vi "CTRE_CANTalonSRX_ConfigEnabledLimits.vi"(0 "CAN Talon SRX Ref":T1={"DeviceStatus"={"status"=FALSE, "code"=0, "source"=""}, "Type"=enum."PWM", "PWM"={"PWM Channel"=enum."PWM 1", "DeadBand"={"Name"="", "maxPositivePwm"=0, "minPositivePwm"=0, "centerPwm"=0, "maxNegativePwm"=0, "minNegativePwm"=0, "angularRange"=0}}, "CAN"={"Device Number"=0, "SetOutput VI Ref"=variant(enum8{"Percent VBus", "Current", "Speed", "Position", "Voltage"} enum."Percent VBus"), "GetOutput VI Ref"=variant(refnum<k1> refnum), "Enable VI Ref"=variant(dbl 12.0), "Disable VI Ref"=variant(enum8{"Percent VBus", "Speed", "Position", "Slave", "Unchanged / Invalid", "Voltage Compensation", "Current", "Motion Profile"} enum."Percent VBus"), "Data"=variant}, "Invert"=FALSE}, 5 "Override Limit Switches":bool, 7 "Forward Limit Switch Enable":bool=TRUE, 9 "Reverse Limit Switch Enable":bool=TRUE, 11 "error in (no error)":errorcluster, 12 "Forward Soft Limit Enable":bool, 13 "Reverse Soft Limit Enable":bool) -> (4 "CAN Talon SRX Ref":T1={"DeviceStatus"={"status"=FALSE, "code"=0, "source"=""}, "Type"=enum."PWM", "PWM"={"PWM Channel"=enum."PWM 1", "DeadBand"={"Name"="", "maxPositivePwm"=0, "minPositivePwm"=0, "centerPwm"=0, "maxNegativePwm"=0, "minNegativePwm"=0, "angularRange"=0}}, "CAN"={"Device Number"=0, "SetOutput VI Ref"=variant(enum8{"Percent VBus", "Current", "Speed", "Position", "Voltage"} enum."Percent VBus"), "GetOutput VI Ref"=variant(refnum<k1> refnum), "Enable VI Ref"=variant(dbl 12.0), "Disable VI Ref"=variant(enum8{"Percent VBus", "Speed", "Position", "Slave", "Unchanged / Invalid", "Voltage Compensation", "Current", "Motion Profile"} enum."Percent VBus"), "Data"=variant}, "Invert"=FALSE}, 15 "error out":errorcluster)   [LabVIEW 2016]
doc: "Configure the enable state of the hardware limit switches and the soft limits."
uses:
  <vilib>/Rock Robotics/WPI/MotorControl/WPI_MotorControlDeviceRef.ctl
  <vilib>/Rock Robotics/WPI/MotorControl/WPI_MotorControlType.ctl
  <vilib>/Rock Robotics/SystemInterfaces/DIO/FPGA_DIOPWMChannel.ctl
  <vilib>/Rock Robotics/WPI/PWM/WPI_PWMDeadband.ctl
  <vilib>/Rock Robotics/WPI/ThirdParty/CanMotor/CTRLib-LV-TalonSRX/CTRE_CANTalonSRX_Params.ctl
  <vilib>/Rock Robotics/WPI/ThirdParty/CanMotor/CTRLib-LV-TalonSRX/CTRE_CANTalonSRX_UsageTypes.ctl
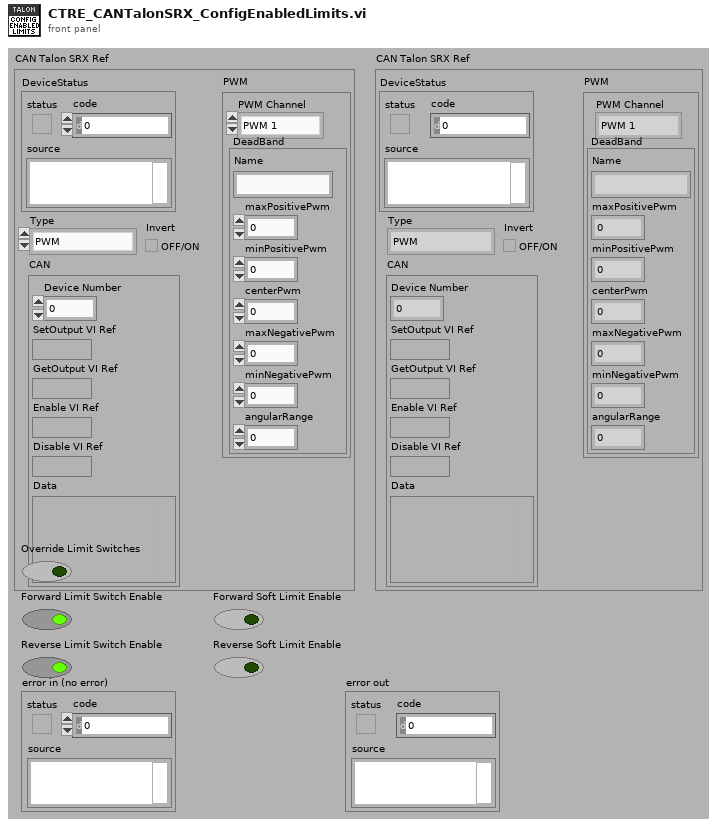
[diagram p1: front panel]
types:
  T1 = typedef "WPI_MotorControlDeviceRef.ctl" = cluster{"DeviceStatus":errorcluster, "Type":T2, "PWM":cluster{"PWM Channel":T3, "DeadBand":T4}, "CAN":cluster{"Device Number":u8, "SetOutput VI Ref":variant, "GetOutput VI Ref":variant, "Enable VI Ref":variant, "Disable VI Ref":variant, "Data":variant}, "Invert":bool}
  T2 = typedef "WPI_MotorControlType.ctl" = enum16{"PWM", "CAN"}
  T3 = typedef "FPGA_DIOPWMChannel.ctl" = enum8{"PWM 0", "PWM 1", "PWM 2", "PWM 3", "PWM 4", "PWM 5", "PWM 6", "PWM 7", "PWM 8", "PWM 9", "PWM MXP 0", "PWM MXP 1", "PWM MXP 2", "PWM MXP 3", "PWM MXP 4", "PWM MXP 5", "PWM MXP 6", "PWM MXP 7", "PWM MXP 8", "PWM MXP 9", "Invalid"}
  T4 = typedef "WPI_PWMDeadband.ctl" = cluster{"Name":string, "maxPositivePwm":i32, "minPositivePwm":i32, "centerPwm":i32, "maxNegativePwm":i32, "minNegativePwm":i32, "angularRange":u16}
  T5 = typedef "CTRE_CANTalonSRX_Params.ctl" = u8
  T6 = typedef "CTRE_CANTalonSRX_UsageTypes.ctl" = u32
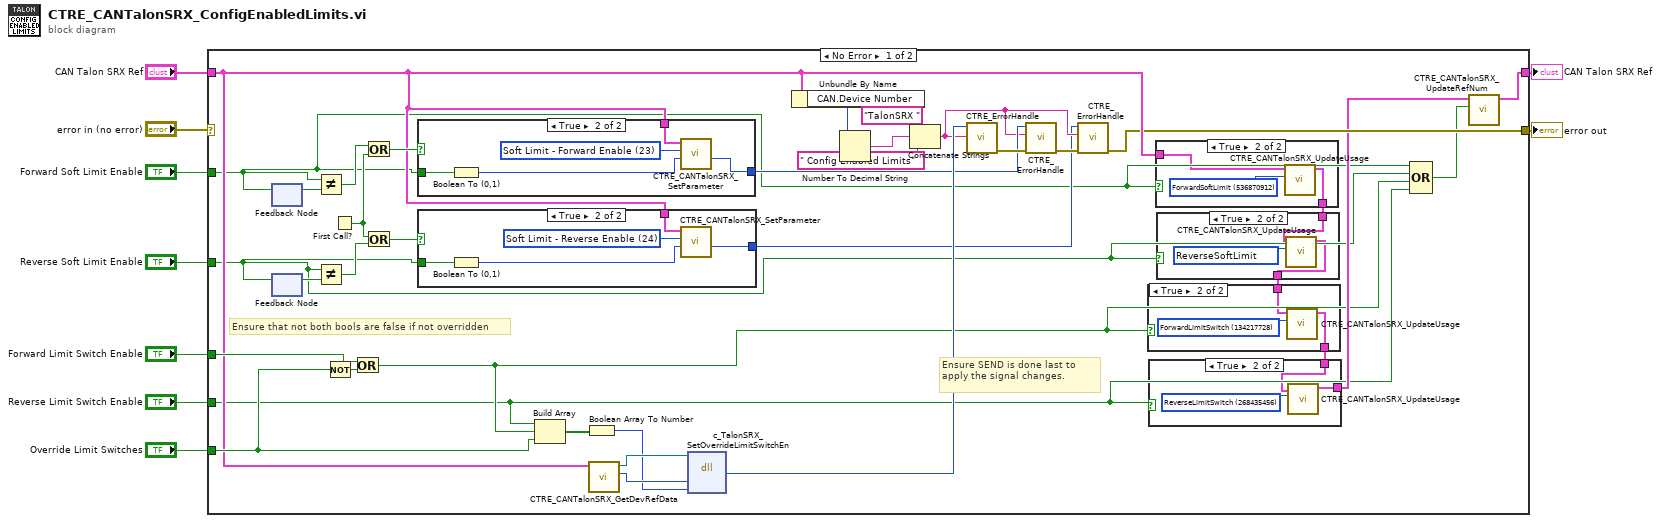
[diagram p0: block diagram]
diagram:
  n1 = case shown="No Error" "error in (no error)" {
    selector: "error in (no error)" -> [_ w73]
    tunnel: [w20 w73] -> w9
    tunnel: [w19 w72] -> w7
    tunnel: "CAN Talon SRX Ref" -> [w27 w72]
    tunnel: "Reverse Soft Limit Enable" -> [w13 _]
    tunnel: "Forward Soft Limit Enable" -> [w14 _]
    tunnel: "Reverse Limit Switch Enable" -> [w11 _]
    tunnel: "Forward Limit Switch Enable" -> [w37 _]
    tunnel: "Override Limit Switches" -> [w36 _]
    frame No Error {
      # "Ensure that not both bools are false if not overridden"
      # "Ensure SEND is done last to apply the signal changes."
      n2 = feedback #1() -> (w41:bool)  [unwired: 1 in]
      n3 = feedback-in #1(w14) -> ()
      n4 = feedback-in #2(w13) -> ()
      n5 = feedback #2() -> (w45:bool)  [unwired: 1 in]
      n6 = Not Equal?(x=w14, y=w41) -> (x != y?=w42:bool)
      n7 = Not Equal?(x=w13, y=w45) -> (x != y?=w43:bool)
      n8 = Not(x=w36) -> (.not. x?=w38:bool)
      n9 = First Call?() -> (First Call?: T/F=w40:bool)
      n10 = Or(x=w37, y=w38) -> (x .or. y?=w12:bool)
      n11 = Or(x=w42, y=w40) -> (x .or. y?=w39:bool)
      n12 = Or(x=w40, y=w43) -> (x .or. y?=w44:bool)
      n13 = case shown="True" w39 {
        tunnel: w14 -> [_ w65]
        tunnel: w27 -> [_ w63]
        tunnel: [_ w62] -> w24
        frame False {
        }
        frame True {
          w66 = T5 23 items=["Slot 0 - P"=1, "Slot 0 - I"=2, "Slot 0 - D"=3, "Slot 0 - F"=4, "Slot 0 - I Zone"=5, "Slot 0 - Ramp Rate"=6, "Slot 1 - P"=11, "Slot 1 - I"=12, "Slot 1 - D"=13, "Slot 1 - F"=14, "Slot 1 - I Zone"=15, "Slot 1 - Ramp Rate"=16, "Soft Limit - Forward"=21, "Soft Limit - Reverse"=22, "Soft Limit - Forward Enable"=23, "Soft Limit - Reverse Enable"=24, "On Boot - Brake Mode"=31, "On Boot - Limit Normally Closed - Forward"=32, "On Boot - Limit Normally Closed - Reverse"=33, "On Boot - Limit Disabled - Forward"=34, "On Boot - Limit Disabled - Reverse"=35, "Fault - Over Temp"=41, "Fault - Under Voltage"=42, "Fault - Forward Limit"=43, "Fault - Reverse Limit"=44, "Fault - Hardware Failure"=45, "Fault - Forward Soft Limit"=46, "Fault - Reverse Soft Limit"=47, "Sticky Fault - Over Temp"=48, "Sticky Fault - Under Voltage"=49, "Sticky Fault - Forward Limit"=50, "Sticky Fault - Reverse Limit"=51, "Sticky Fault - Forward Soft Limit"=52, "Sticky Fault - Reverse Soft Limit"=53, "Applied Throttle"=61, "Closed-Loop Error"=62, "Select Feedback Device"=63, "Reverse Closed-Loop Output"=64, "Mode Select"=65, "Profile Slot Select"=66, "Ramp Throttle"=67, "Reverse Feedback Sensor"=68, "Limit Switch Enabled"=69, "Limit Switch Closed - Forward"=70, "Limit Switch Closed - Reverse"=71, "Sensor Position"=73, "Sensor Velocity"=74, "Current"=75, "Brake is Enabled"=76, "Encoder Position"=77, "Encoder Velocity"=78, "Encoder Index Rise Events"=79, "Encoder A Pin State"=80, "Encoder B Pin State"=81, "Encoder Index Pin State"=82, "Analog In with Overflow"=83, "Analog In Velocity"=84, "Temperature"=85, "Battery Voltage"=86, "Reset Count"=87, "Reset Flags"=88, "Firmware Version"=89, "Settings Changed"=90] ("Parameter")
          n14 = Boolean To (0,1)(Boolean=w65) -> (0, 1=w64:i16)
          n15 = call <vilib>:"CTRE_CANTalonSRX_SetParameter.vi"("Value"=w64, "Parameter"=w66, "CAN Talon SRX Ref"=w63) -> ("Error Code"=w62:i32)  [unwired: 6 in, 2 out]
        }
      }
      n16 = case shown="True" w44 {
        tunnel: w13 -> [_ w70]
        tunnel: w27 -> [_ w68]
        tunnel: [_ w67] -> w21
        frame False {
        }
        frame True {
          w71 = T5 24 items=["Slot 0 - P"=1, "Slot 0 - I"=2, "Slot 0 - D"=3, "Slot 0 - F"=4, "Slot 0 - I Zone"=5, "Slot 0 - Ramp Rate"=6, "Slot 1 - P"=11, "Slot 1 - I"=12, "Slot 1 - D"=13, "Slot 1 - F"=14, "Slot 1 - I Zone"=15, "Slot 1 - Ramp Rate"=16, "Soft Limit - Forward"=21, "Soft Limit - Reverse"=22, "Soft Limit - Forward Enable"=23, "Soft Limit - Reverse Enable"=24, "On Boot - Brake Mode"=31, "On Boot - Limit Normally Closed - Forward"=32, "On Boot - Limit Normally Closed - Reverse"=33, "On Boot - Limit Disabled - Forward"=34, "On Boot - Limit Disabled - Reverse"=35, "Fault - Over Temp"=41, "Fault - Under Voltage"=42, "Fault - Forward Limit"=43, "Fault - Reverse Limit"=44, "Fault - Hardware Failure"=45, "Fault - Forward Soft Limit"=46, "Fault - Reverse Soft Limit"=47, "Sticky Fault - Over Temp"=48, "Sticky Fault - Under Voltage"=49, "Sticky Fault - Forward Limit"=50, "Sticky Fault - Reverse Limit"=51, "Sticky Fault - Forward Soft Limit"=52, "Sticky Fault - Reverse Soft Limit"=53, "Applied Throttle"=61, "Closed-Loop Error"=62, "Select Feedback Device"=63, "Reverse Closed-Loop Output"=64, "Mode Select"=65, "Profile Slot Select"=66, "Ramp Throttle"=67, "Reverse Feedback Sensor"=68, "Limit Switch Enabled"=69, "Limit Switch Closed - Forward"=70, "Limit Switch Closed - Reverse"=71, "Sensor Position"=73, "Sensor Velocity"=74, "Current"=75, "Brake is Enabled"=76, "Encoder Position"=77, "Encoder Velocity"=78, "Encoder Index Rise Events"=79, "Encoder A Pin State"=80, "Encoder B Pin State"=81, "Encoder Index Pin State"=82, "Analog In with Overflow"=83, "Analog In Velocity"=84, "Temperature"=85, "Battery Voltage"=86, "Reset Count"=87, "Reset Flags"=88, "Firmware Version"=89, "Settings Changed"=90] ("Parameter")
          n17 = Boolean To (0,1)(Boolean=w70) -> (0, 1=w69:i16)
          n18 = call <vilib>:"CTRE_CANTalonSRX_SetParameter.vi"("Value"=w69, "Parameter"=w71, "CAN Talon SRX Ref"=w68) -> ("Error Code"=w67:i32)  [unwired: 6 in, 2 out]
        }
      }
      n19 = Build Array(w11, w12, w36) -> (w33:bool[])
      n20 = Boolean Array To Number(Boolean array=w33) -> (number=w32:u8)
      n21 = call <vilib>:"CTRE_CANTalonSRX_GetDevRefData.vi"("MotorControlDevRef"=w27) -> ("handle"=w34:u64, "Library"=w35:path)  [unwired: 6 in, 3 out]
      n22 = dll-call lib="?" fn="c_TalonSRX_SetOverrideLimitSwitchEn"(path in=w35, "handle"=w34, "param"=w32) -> ("return type"=w26:i32)  [unwired: 4 in, 2 out]
      n23 = Unbundle By Name(w27) -> ("CAN.Device Number"=w28:u8)
      n24 = Number To Decimal String(number=w28) -> (decimal integer string=w30:string)  [unwired: 1 in]
      n25 = Concatenate Strings("TalonSRX " ("string"), w30, " Config Enabled Limits" ("string")) -> (w22:string)
      n26 = call <vilib>:"CTRE_ErrorHandle.vi"("origin"=w22, "code"=w26) -> ("error out"=w25:errorcluster)  [unwired: 9 in]
      n27 = call <vilib>:"CTRE_ErrorHandle.vi"("error in"=w25, "origin"=w22, "code"=w24) -> ("error out"=w23:errorcluster)  [unwired: 8 in]
      n28 = call <vilib>:"CTRE_ErrorHandle.vi"("error in"=w23, "origin"=w22, "code"=w21) -> ("error out"=w20:errorcluster)  [unwired: 8 in]
      n29 = case shown="True" w14 {
        tunnel: w27 -> [w58 w61]
        tunnel: [w58 w59] -> w18
        frame False {
        }
        frame True {
          w60 = T6 536870912 items=["Default"=0, "PercentVbus"=1, "Position"=2, "Speed"=4, "Current"=8, "Voltage"=16, "Follower"=32, "MotionProfile"=64, "MotionMagic"=128, "VRampRate"=4194304, "CurrentLimit"=8388608, "ZeroSensorI"=16777216, "ZeroSensorF"=33554432, "ZeroSensorR"=67108864, "ForwardLimitSwitch"=134217728, "ReverseLimitSwitch"=268435456, "ForwardSoftLimit"=536870912, "ReverseSoftLimit"=1073741824, "MultiProfile"=2147483648] ("Usage")
          n30 = call <vilib>:"CTRE_CANTalonSRX_UpdateUsage.vi"("Usage"=w60, "CAN Talon SRX Ref"=w61) -> ("CAN Talon SRX"=w59:T1)  [unwired: 8 in, 1 out]
        }
      }
      n31 = case shown="True" w13 {
        tunnel: w18 -> [w54 w56]
        tunnel: [w54 w55] -> w17
        frame False {
        }
        frame True {
          w57 = T6 1073741824 items=["Default"=0, "PercentVbus"=1, "Position"=2, "Speed"=4, "Current"=8, "Voltage"=16, "Follower"=32, "MotionProfile"=64, "MotionMagic"=128, "VRampRate"=4194304, "CurrentLimit"=8388608, "ZeroSensorI"=16777216, "ZeroSensorF"=33554432, "ZeroSensorR"=67108864, "ForwardLimitSwitch"=134217728, "ReverseLimitSwitch"=268435456, "ForwardSoftLimit"=536870912, "ReverseSoftLimit"=1073741824, "MultiProfile"=2147483648] ("Usage")
          n32 = call <vilib>:"CTRE_CANTalonSRX_UpdateUsage.vi"("Usage"=w57, "CAN Talon SRX Ref"=w56) -> ("CAN Talon SRX"=w55:T1)  [unwired: 8 in, 1 out]
        }
      }
      n33 = case shown="True" w12 {
        tunnel: w17 -> [w50 w52]
        tunnel: [w50 w51] -> w16
        frame False {
        }
        frame True {
          w53 = T6 134217728 items=["Default"=0, "PercentVbus"=1, "Position"=2, "Speed"=4, "Current"=8, "Voltage"=16, "Follower"=32, "MotionProfile"=64, "MotionMagic"=128, "VRampRate"=4194304, "CurrentLimit"=8388608, "ZeroSensorI"=16777216, "ZeroSensorF"=33554432, "ZeroSensorR"=67108864, "ForwardLimitSwitch"=134217728, "ReverseLimitSwitch"=268435456, "ForwardSoftLimit"=536870912, "ReverseSoftLimit"=1073741824, "MultiProfile"=2147483648] ("Usage")
          n34 = call <vilib>:"CTRE_CANTalonSRX_UpdateUsage.vi"("Usage"=w53, "CAN Talon SRX Ref"=w52) -> ("CAN Talon SRX"=w51:T1)  [unwired: 8 in, 1 out]
        }
      }
      n35 = case shown="True" w11 {
        tunnel: w16 -> [w46 w48]
        tunnel: [w46 w47] -> w15
        frame False {
        }
        frame True {
          w49 = T6 268435456 items=["Default"=0, "PercentVbus"=1, "Position"=2, "Speed"=4, "Current"=8, "Voltage"=16, "Follower"=32, "MotionProfile"=64, "MotionMagic"=128, "VRampRate"=4194304, "CurrentLimit"=8388608, "ZeroSensorI"=16777216, "ZeroSensorF"=33554432, "ZeroSensorR"=67108864, "ForwardLimitSwitch"=134217728, "ReverseLimitSwitch"=268435456, "ForwardSoftLimit"=536870912, "ReverseSoftLimit"=1073741824, "MultiProfile"=2147483648] ("Usage")
          n36 = call <vilib>:"CTRE_CANTalonSRX_UpdateUsage.vi"("Usage"=w49, "CAN Talon SRX Ref"=w48) -> ("CAN Talon SRX"=w47:T1)  [unwired: 8 in, 1 out]
        }
      }
      n37 = Compound Arithmetic op=OR(w14, w13, w12, w11) -> (w10:bool)
      n38 = call <vilib>:"CTRE_CANTalonSRX_UpdateRefNum.vi"("Update"=w10, "CAN Talon SRX Ref"=w15) -> ("CAN Talon SRX Ref"=w19:T1)  [unwired: 9 in]
    }
    frame Error {
    }
  }
  "CAN Talon SRX Ref" <- w7
  "error out" <- w9
